vi "write all relays.vi"(8 "error in (no error)":errorcluster, 11 "USB IO in":refnum<class "USB IO.lvclass">) -> (0 "error out":errorcluster, 3 "USB IO out":refnum<class "USB IO.lvclass">)   [LabVIEW 2025, in "USB IO.lvclass"]
uses:
  USB IO.lvclass
  USB IO.lvclass/USB IO.ctl
  <vilib>/DAQmx/write.llb/DAQmx Write (Digital 1D Bool NChan 1Samp 1Line).vi
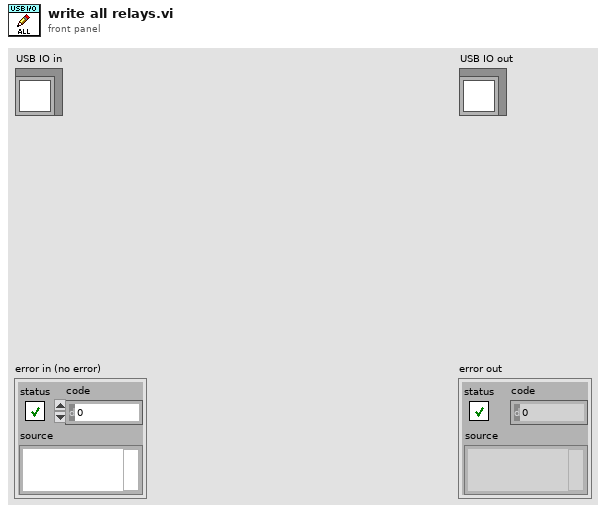
[diagram p1: front panel]
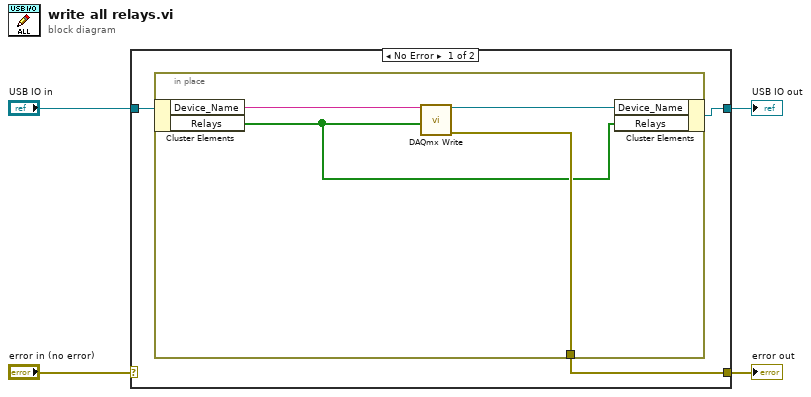
[diagram p0: block diagram]
diagram:
  n1 = case shown="No Error" "error in (no error)" {
    selector: "error in (no error)" -> [_ w13]
    tunnel: [w6 w13] -> w3
    tunnel: [w5 w12] -> w1
    tunnel: "USB IO in" -> [w7 w12]
    frame No Error {
      n2 = in-place {
        in-place-border: [w9] -> w6
        n3 = in-place-cluster #1(w7) -> ("Device_Name"=w11:string, "Relays"=w8:bool[])
        n4 = call-poly <vilib>:"DAQmx Write.vi"("task/channels in"=w11, "data"=w8) -> ("task out"=w10:refnum<k21>, "error out"=w9:errorcluster)  [unwired: 11 in, 1 out]
        n5 = in-place-cluster #1("Device_Name"=w10, "Relays"=w8) -> (w5:refnum<class "USB IO.lvclass">)
      }
    }
    frame Error {
    }
  }
  "error out" <- w3
  "USB IO out" <- w1
